vi "New.vi"(11 "max file size [MB](50)":dbl=50.0) -> (3 "size trigger":refnum<class "RolloverTrigger.Size.lvclass">)   [LabVIEW 2018, in "GLog.lvlib" / "RolloverTrigger.Size.lvclass"]
doc: "Creates a new rollover trigger based on a maximum file size.\n\nIf \"max file size\" is 0, the file will never rollover."
uses:
  RolloverTrigger.Size.lvclass
  RolloverTrigger.Size.lvclass/RolloverTrigger.Size.ctl
panel:
  # "Connector Pane"
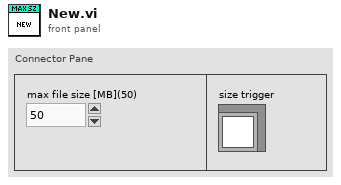
[diagram p1: front panel]
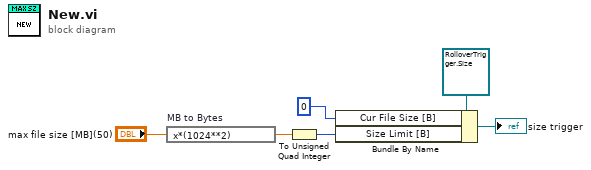
[diagram p0: block diagram]
diagram:
  n1 = expression code="x*(1024**2)" "MB to Bytes"("max file size [MB](50)") -> (w4:dbl)
  n2 = To Unsigned Quad Integer(1:w4) -> (0:w2:u64)
  n3 = Bundle By Name(cluster=refnum<class "RolloverTrigger.Size.lvclass"> refnum ("RolloverTrigger.Size in"), "Cur File Size [B]"=i64 0, "Size Limit [B]"=w2) -> (→"size trigger":refnum<class "RolloverTrigger.Size.lvclass">)
